vi "CLAHE (OpenCV).vi"() -> ()   [LabVIEW 2023]
uses:
  Images/_Images.ctl
panel:
  out "Execution Time, ms":u32
  out "Original":T1(plugin-control)
  in  "Image":T2
  in  "Lock":bool=TRUE
  in  "stop":bool
  in  "Tile Height":i32(slide)=5 scale=1.0..100.0
  in  "Tile Width":i32(slide)=5 scale=1.0..100.0
  in  "Clip Limit":dbl(slide)=40.0 scale=1.0..1000.0
  out "Enhanced":T1(plugin-control)
  # "Contrast Limited Adaptive Histogram Equalization"
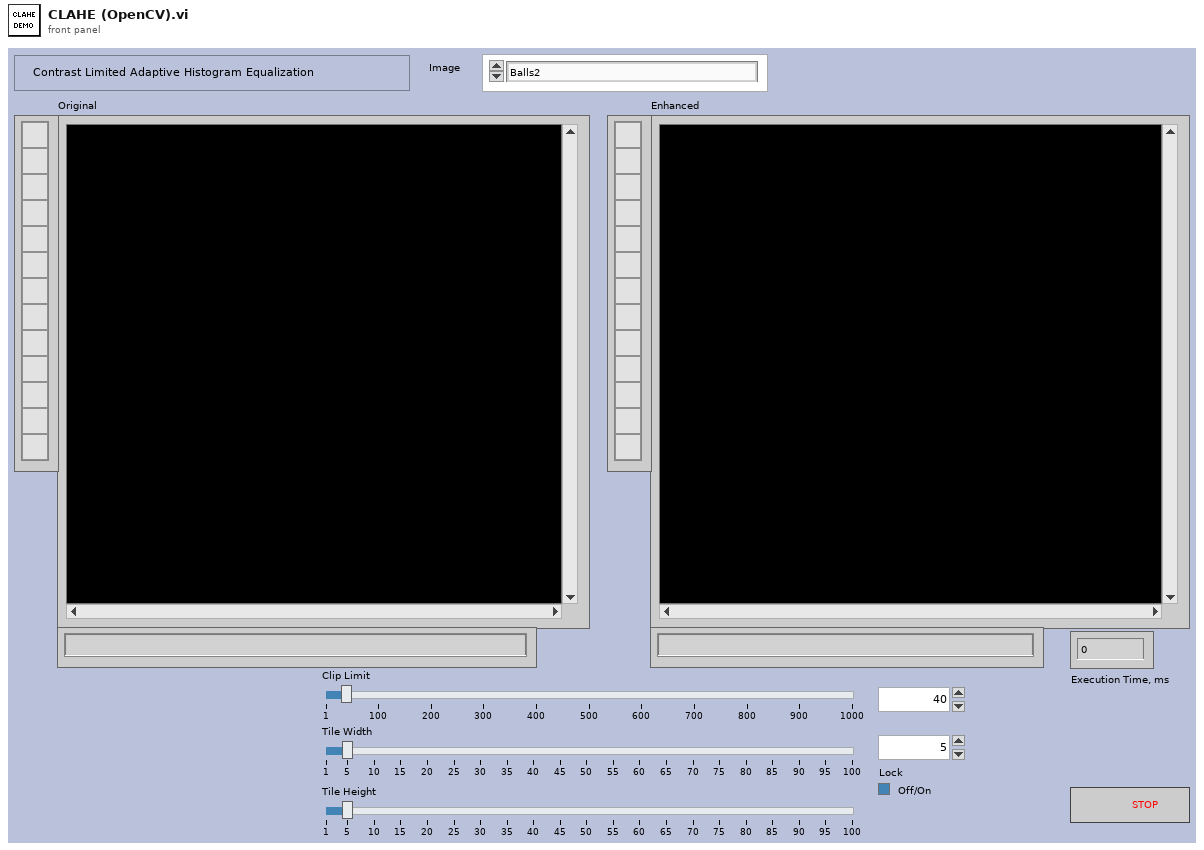
[diagram p1: front panel]
types:
  T1 = typedef "IMAQ Image.ctl" = refnum<image>
  T2 = typedef "_Images.ctl" = enum16{"Balls2", "Battery1", "Battery2", "Connector1", "Subwoofer1", "Subwoofer2", "Subwoofer3", "Subwoofer4", "Hase1", "Lamp1", "Lamp2", "Mouse1", "PhotoLens1", "Po1", "PowerSupply1", "Router", "--- Step Wedges ---", "Stepwedge1", "Stepwedge2", "Stepwedge3", "--- Fusion ---", "Fusion160kV", "Fusion2-120kV", "Fusion2-320kV", "Fusion300kV", "FusionPart1-120kV", "FusionPart1-180kV", "--- PART 01 ---", "Part1", "Part2", "Part3", "Part4", "Part5", "Part6", "Part7", "Part8", "--- Different Integrations ---", "Step2737-02Int", "Step2737-04Int", "Step2737-08Int", "Step2737-16Int", "Step2737-32Int", "Step2737-64Int"}
  T3 = typedef "Image Type" = u32
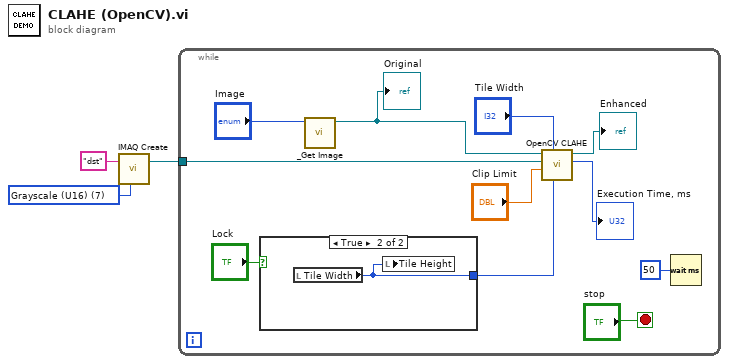
[diagram p0: block diagram]
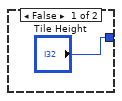
[diagram p2: hidden frame]
diagram:
  w2 = T3 7 items=["Grayscale (U8)", "Grayscale (I16)", "Grayscale (SGL)", "Complex (CSG)", "RGB (U32)", "HSL (U32)", "RGB (U64)", "Grayscale (U16)"] ("Image Type")
  n1 = call "IMAQ Create"("Image Name"="dst", "Image Type"=w2) -> ("New Image"=w1:T1)  [unwired: 3 in, 1 out]
  n2 = while {
    tunnel: w1 -> [w6]
    stop <- "stop" stop-if-true
    n3 = case shown="True" "Lock" {
      tunnel: ["Tile Height" w16] -> w8
      frame False {
      }
      frame True {
        n4 = local read "Tile Width"() -> (w16:i32)
        n5 = local write "Tile Height"(w16) -> ()
      }
    }
    n6 = call "_Get Image.vi"("Image"="Image") -> ("Image Out"=w4:T1)  [unwired: 7 in, 3 out]
    "Original" <- w4
    n7 = call "OpenCV CLAHE.vi"("tileHeight"=w8, "tileWidth"="Tile Width", "ClipLimit"="Clip Limit", "Image Dst"=w6, "Image Src"=w4) -> ("Execution Time, ms"=→"Execution Time, ms":u32, "Image Dst Out"=→"Enhanced":T1)  [unwired: 1 in, 4 out]
    n8 = Wait (ms)(milliseconds to wait=u32 50) -> ()  [unwired: 1 out]
  }
